vi "DAC Configure FP View.vi"(8 "error in":errorcluster, 11 "DAC HeatFlow AIV in":refnum<class "DAC HeatFlow AIV.lvclass">) -> (0 "error out":errorcluster, 3 "DAC HeatFlow AIV out":refnum<class "DAC HeatFlow AIV.lvclass">)   [LabVIEW 2019, in "DAC.lvlib" / "DAC HeatFlow AIV.lvclass"]
uses:
  DAC HeatFlow AIV.lvclass
  C:/Users/wg/Documents/LV_Projects/test-stand/App/DAC/DAC.lvclass
  Results/Results Method.ctl
  Results/DeepU Results/DeepU Results.lvclass
  DAC.lvclass/DAC.ctl
  DAC HeatFlow AIV.lvclass/DAC HeatFlow AIV.ctl
  Results/Results.lvlib
  DAC.lvclass
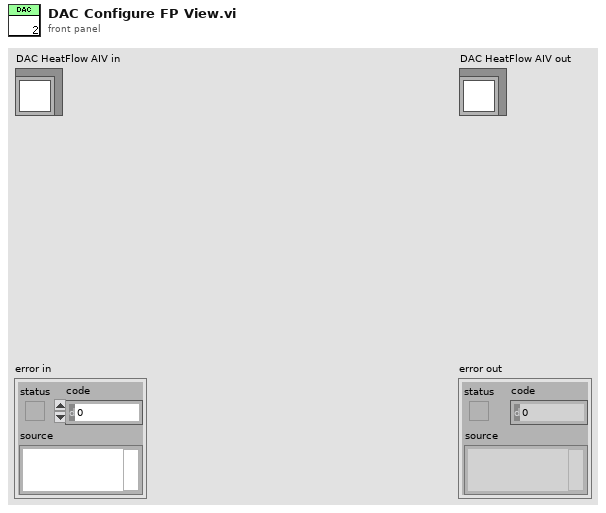
[diagram p1: front panel]
types:
  T1 = typedef "Results.lvlib/Results Method.ctl" = enum16{"Get", "Set"}
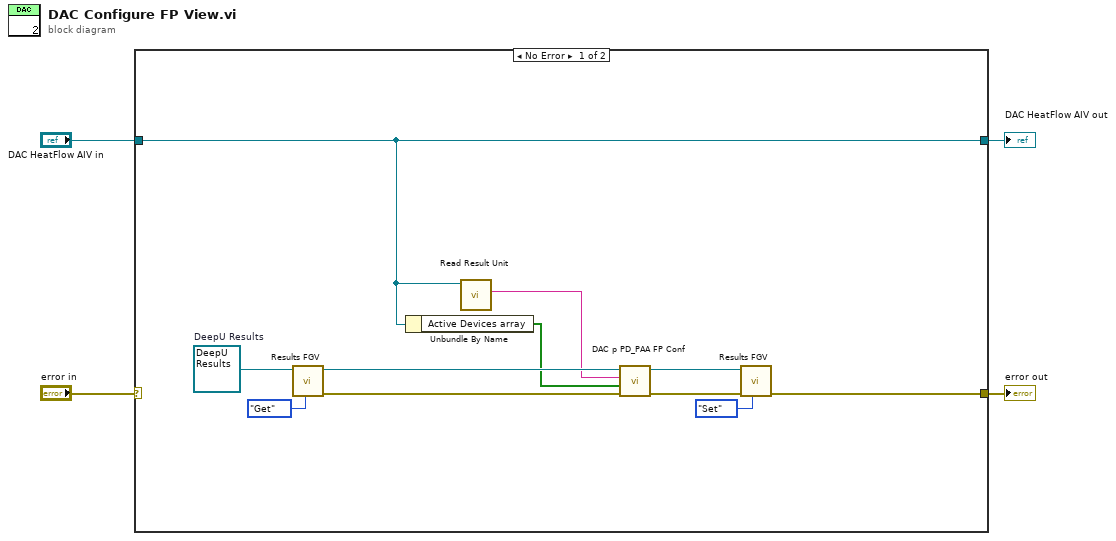
[diagram p0: block diagram]
diagram:
  n1 = case shown="No Error" "error in" {
    selector: "error in" -> [_ w17]
    tunnel: [w15 w17] -> w1
    tunnel: [w11 w16] -> w2
    tunnel: "DAC HeatFlow AIV in" -> [w11 w16]
    frame No Error {
      w14 = refnum<class "DeepU Results.lvclass"> refnum  # DeepU Results
      n2 = call-dynamic "Results FGV.vi"("Method"=Results_Method."Get", "DeepU Results in"=w14) -> ("error out"=w8:errorcluster, "DeepU Results out"=w7:refnum<class "DeepU Results.lvclass">)  [unwired: 8 in]
      n3 = Unbundle By Name(w11) -> ("Active Devices array"=w5:bool[])
      n4 = call "Read Result Unit.vi"("DAC in"=w11) -> ("Unit"=w6:string)  [unwired: 8 in, 2 out]
      n5 = call "DAC p PD_PAA FP Conf.vi"("error in (no error)"=w8, "Used p PD_PAA"=w5, "Result Unit"=w6, "DeepU Results in"=w7) -> ("error out"=w9:errorcluster, "DeepU Results out"=w10:refnum<class "DeepU Results.lvclass">)  [unwired: 6 in]
      n6 = call-dynamic "Results FGV.vi"("Method"=Results_Method."Set", "error in"=w9, "DeepU Results in"=w10) -> ("error out"=w15:errorcluster)  [unwired: 7 in, 1 out]
    }
    frame Error {
    }
  }
  "error out" <- w1
  "DAC HeatFlow AIV out" <- w2
